vi "Service for Authentication.vi"(11 "HTTP Request":refnum<class "HTTP Request.lvclass">) -> (2 "Service for Authentication":string)   [LabVIEW 2015, in "NI_AWS_Core.lvlib" / "HTTP Request.lvclass"]
uses:
  HTTP Request.lvclass
  HTTP Request.lvclass/HTTP Request.ctl
  Read Service.vi
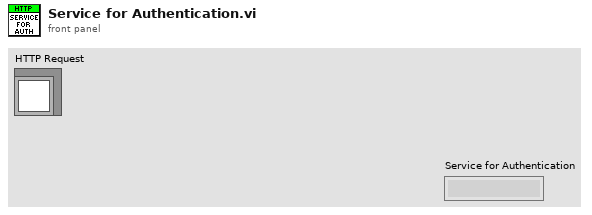
[diagram p1: front panel]
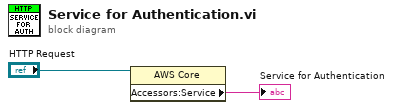
[diagram p0: block diagram]
diagram:
  n1 = property class="AWS Core"(reference="HTTP Request") -> ("Accessors:Service"=→"Service for Authentication":string)  [unwired: 1 in, 2 out]
